vi "Scale deg To arcsec.vi"() -> ()   [LabVIEW 2015, in "Utility.lvlib"]
uses:
  Utility.lvlib
panel:
  out "arcsec":dbl
  in  "deg":dbl
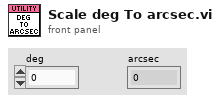
[diagram p1: front panel]
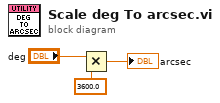
[diagram p0: block diagram]
diagram:
  n1 = Multiply(x="deg", y=3600.0) -> (x*y=→"arcsec":dbl)
